vi "Clear.vi"(8 "error in (no error)":errorcluster, 11 "Execution API In":refnum<class "Execution API.lvclass">) -> (0 "error out":errorcluster, 3 "Execution API Out":refnum<class "Execution API.lvclass">)   [LabVIEW 2020, in "Execution API.lvclass"]
doc: "Clears any resorces allocated during initialization."
uses:
  Execution API.lvclass
  Execution API.lvclass/Execution API.ctl
  Test Runner/Test Runner.lvclass
  Report Generator/Report Generator.lvclass
  Result Collector/Result Collector.lvclass
  Application Framework/Process Classes/Process/Process.lvclass
  Helper Classes/Test Finder/Test Finder.lvclass
  Application Framework/Process Classes/Error Handler/Error Handler.lvclass
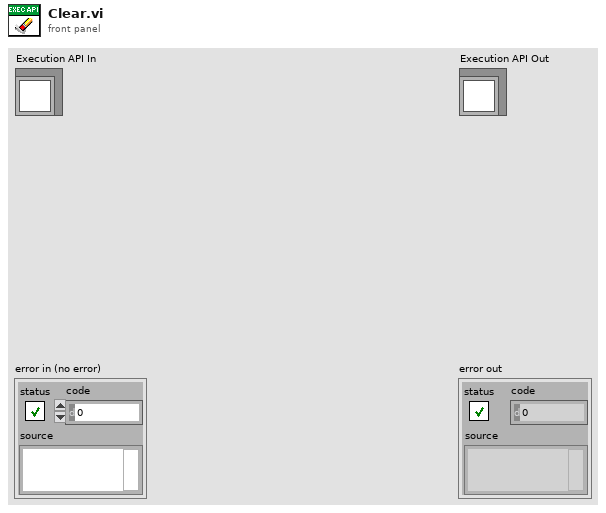
[diagram p1: front panel]
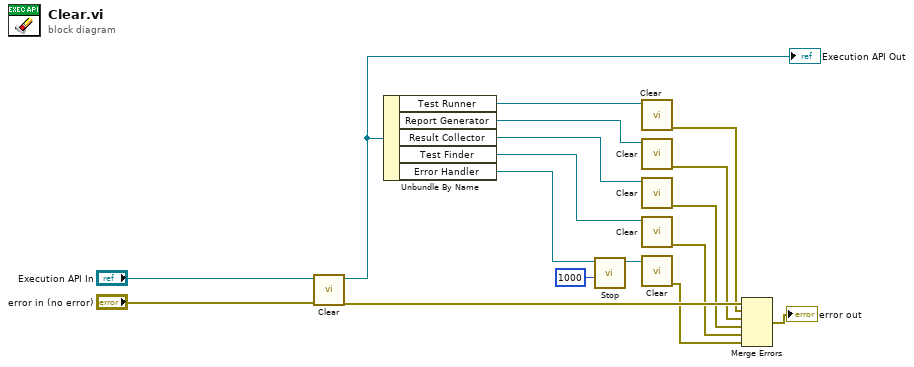
[diagram p0: block diagram]
diagram:
  n1 = call-parent "Clear.vi"("error in (no error)"="error in (no error)", "Process In"="Execution API In") -> ("error out"=w17:errorcluster, "Process Out"=w15:refnum<class "Execution API.lvclass">)  [unwired: 8 in]
  "Execution API Out" <- w15
  n2 = Unbundle By Name(w15) -> ("Test Runner"=w14:refnum<class "Test Runner.lvclass">, "Report Generator"=w13:refnum<class "Report Generator.lvclass">, "Result Collector"=w9:refnum<class "Result Collector.lvclass">, "Test Finder"=w7:refnum<class "Test Finder.lvclass">, "Error Handler"=w3:refnum<class "Error Handler.lvclass">)
  n3 = call-dynamic "Stop.vi"("timeout in ms (-1)"=1000, "Process In"=w3) -> ("Process Out"=w2:refnum<class "Error Handler.lvclass">)  [unwired: 7 in, 2 out]
  n4 = call-dynamic "Clear.vi"("Test Runner In"=w14) -> ("error out"=w11:errorcluster)  [unwired: 9 in, 1 out]
  n5 = call-dynamic "Clear.vi"("Process In"=w13) -> ("error out"=w10:errorcluster)  [unwired: 9 in, 1 out]
  n6 = call-dynamic "Clear.vi"("Report Generator In"=w9) -> ("error out"=w8:errorcluster)  [unwired: 9 in, 1 out]
  n7 = call "Clear.vi"("Test Finder in"=w7) -> ("error out"=w6:errorcluster)  [unwired: 9 in, 1 out]
  n8 = call-dynamic "Clear.vi"("Error Handler In"=w2) -> ("error out"=w1:errorcluster)  [unwired: 9 in, 1 out]
  n9 = Merge Errors(w17, w11, w10, w8, w6, w1) -> (→"error out":errorcluster)
